vi "Miso Logic 64-bit.vi"(0 "MISO":bool, 5 "sample MISO":bool, 7 "controller interface":T1) -> (4 "read data":u64)   [LabVIEW 2015]
doc: "This VI captures a single bit of MISO data to for the read data word."
uses:
  Controls/Controller Interface.ctl
panel:
  # "This VI captures a single bit of MISO data to for the read data word."
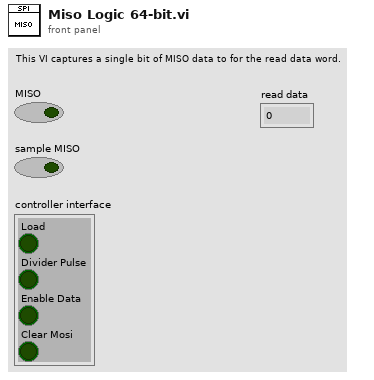
[diagram p1: front panel]
types:
  T1 = typedef "Controller Interface.ctl" = cluster{"Load":bool, "Divider Pulse":bool, "Enable Data":bool, "Clear Mosi":bool}
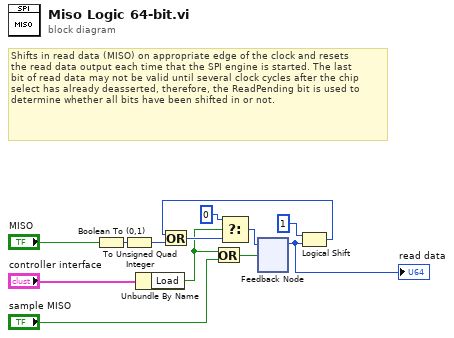
[diagram p0: block diagram]
diagram:
  # "Shifts in read data (MISO) on appropriate edge of the clock and resets\nthe read data output each time that the SPI engine is started. The last\nbit of read data may not be valid until several clock cycles after the chip select has already deasserted, therefore, the ReadPending bit is used to determine whether all bits have been shifted in or not."
  n1 = Boolean To (0,1)(Boolean="MISO") -> (0, 1=w11:i16)
  n2 = To Unsigned Quad Integer(1:w11) -> (0:w9:u64)
  n3 = Unbundle By Name("controller interface") -> ("Load"=w3:bool)
  n4 = Or(x=w3, y="sample MISO") -> (x .or. y?=w7:bool)
  n5 = feedback #1() -> (w12:u64)  [unwired: 1 in]
  "read data" <- w12
  n6 = Logical Shift(y=i16 1, x=w12) -> (x << y=w8:u64)
  n7 = Or(x=w8, y=w9) -> (x .or. y?=w6:u64)
  n8 = Select(t=u64 0, s=w3, f=w6) -> (s? t:f=w5:u64)
  n9 = feedback-in #1(w5, w7) -> ()
